vi "Read Parameters to process.vi"(8 "error in":errorcluster, 11 "GPIC Core runtime in":refnum<class "GPIC Core runtime.lvclass">) -> (0 "error out":errorcluster, 2 "Parameters to process":T1, 3 "GPIC Core runtime out":refnum<class "GPIC Core runtime.lvclass">)   [LabVIEW 2017, in "GPIC Core runtime.lvclass"]
uses:
  GPIC Core runtime.lvclass
  configuration/parameter data indices.ctl
  GPIC Core runtime.lvclass/GPIC Core runtime.ctl
  configuration/GPIC Core configuration.lvclass
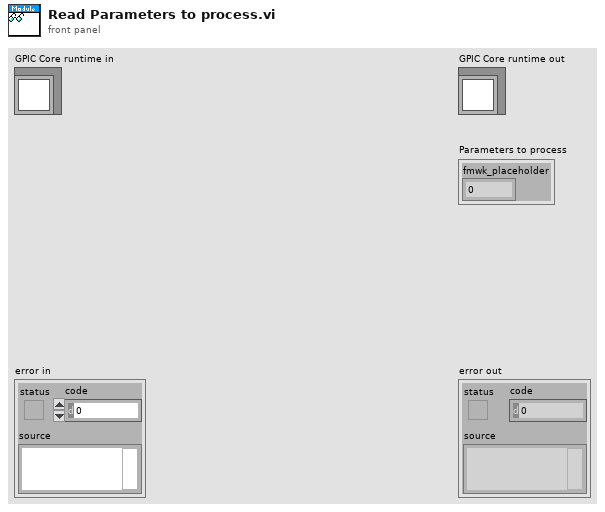
[diagram p1: front panel]
types:
  T1 = typedef "GPIC Core configuration.lvclass/parameter data indices.ctl" = cluster{"fmwk_placeholder":i32}
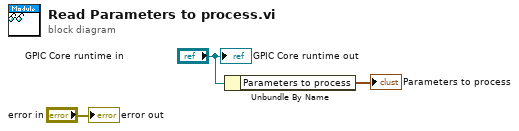
[diagram p0: block diagram]
diagram:
  n1 = Unbundle By Name("GPIC Core runtime in") -> ("Parameters to process"=→"Parameters to process":T1)
  "error out" <- "error in"
  "GPIC Core runtime out" <- "GPIC Core runtime in"
